vi "split4.vi"(4 "error in":errorcluster, 7 "Waveforms":waveform(i16)[](array[waveform])) -> (0 "error out":errorcluster, 1 "detected phase (deg)":dbl, 2 "Sync":waveform(i16), 3 "Array 2":waveform(i16)[][](array[waveform]))   [LabVIEW 2010]
uses:
  <vilib>/measure/matone.llb/Extract Single Tone Information 1 Chan.vi
  <vilib>/measure/NI_MAPro.lvlib
panel:
  out "frequency":dbl format="%.2p"
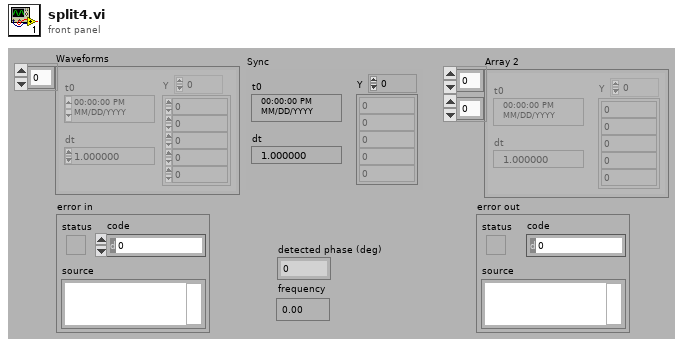
[diagram p1: front panel]
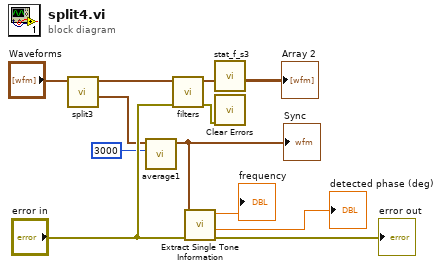
[diagram p0: block diagram]
diagram:
  n1 = call "split3.vi"("Array of Waveform In"="Waveforms") -> ("Sync"=w3:waveform(i16), "Array of Waveform"=w5:waveform(i16)[])  [unwired: 5 in]
  n2 = call "average1.vi"("Size"=3000, "SignalIn"=w3) -> ("output waveform"=w8:waveform(i16))  [unwired: 5 in]
  "Sync" <- w8
  n3 = call "filters.vi"("error in (no error)"="error in", "Array"=w5) -> ("error out"=w1:errorcluster, "Array 2"=w6:waveform(i16)[])  [unwired: 4 in]
  n4 = call-poly <vilib>:"Extract Single Tone Information.vi"("error in (no error)"="error in", "time signal in"=w8) -> ("error out"=→"error out":errorcluster, "detected phase (deg)"=→"detected phase (deg)":dbl, "detected frequency"=→"frequency":dbl)  [unwired: 4 in, 3 out]
  n5 = call "stat_f_s3.vi"("Array of Wfm"=w6) -> ("Array 2"=→"Array 2":waveform(i16)[][])  [unwired: 6 in]
  n6 = call <vilib>:"Clear Errors.vi"("error in (no error)"=w1) -> ()  [unwired: 6 in, 1 out]
